vi "Teleop.vi"(10 "Match Info":T1={"Autonomous Elapsed Seconds"=0.0, "TeleOp Elapsed Seconds"=0.0, "Disabled Elapsed Seconds"=0.0, "Visited Autonomous"=FALSE, "Visited TeleOp"=FALSE, "Visited Disabled"=FALSE, "Autonomous Settings"={"Autonomous Style"=enum."Independent", "VI Refnum"=refnum}}, 11 "Call Context":T2) -> ()   [LabVIEW 2019]
doc: "This VI is called for each TeleOp packet received from the DS where the robot is not disabled. It is often used to read from the joysticks and update I/O or to update setpoints for timed control loops. It should complete and return within 20 milliseconds or it may miss DS packets."
uses:
  <vilib>/Rock Robotics/WPI/DriverStation/WPI_DriverStationDerivedRobotMode.ctl
  <vilib>/Rock Robotics/WPI/DriverStation/WPI_DriverStationMatch Info.ctl
  <vilib>/Rock Robotics/WPI/Utilities/WPI_GetSetVariantRefNum.vi
  <vilib>/Rock Robotics/Network Tables/NT Write Boolean Array.vi
  <vilib>/Rock Robotics/Network Tables/NT Write Numeric Array.vi
  <vilib>/Rock Robotics/Network Tables/NT Read Boolean.vi
  <vilib>/Rock Robotics/Network Tables/NT Read Number.vi
panel:
  out "Sample Slider 0":dbl(slide) scale=0.0..5.0
  out "Sample Boolean 1":bool
  out "Sample Boolean 0":bool
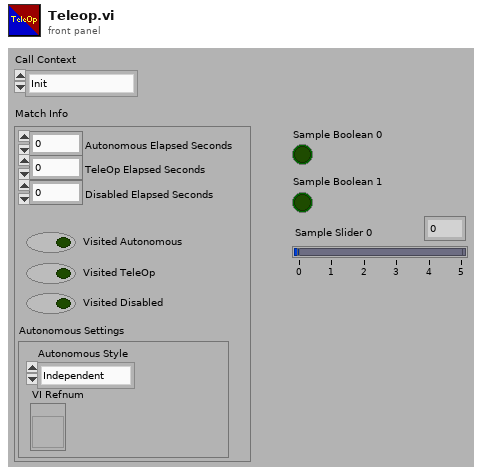
[diagram p1: front panel]
types:
  T1 = typedef "WPI_DriverStationMatch Info.ctl" = cluster{"Autonomous Elapsed Seconds":dbl, "TeleOp Elapsed Seconds":dbl, "Disabled Elapsed Seconds":dbl, "Visited Autonomous":bool, "Visited TeleOp":bool, "Visited Disabled":bool, "Autonomous Settings":cluster{"Autonomous Style":enum16{"Iterative", "Independent"}, "VI Refnum":refnum<vi>}}
  T2 = typedef "WPI_DriverStationDerivedRobotMode.ctl" = enum16{"Init", "Execute", "Stop"}
  T3 = typedef "WPI_JoystickDevRef.ctl" = cluster{"Device":T4}
  T4 = typedef "WPI_JoystickDeviceEnum.ctl" = enum16{"USB 0", "USB 1", "USB 2", "USB 3", "USB 4", "USB 5"}
  T5 = cluster{"Buttons[0]":bool, "Buttons[1]":bool, "Buttons[2]":bool, "Buttons[3]":bool, "Buttons[4]":bool, "Buttons[5]":bool, "Buttons[6]":bool, "Buttons[7]":bool, "Buttons[8]":bool}
  T6 = cluster{"Axes[0]":dbl, "Axes[1]":dbl, "Axes[2]":dbl, "Axes[3]":dbl, "Axes[4]":dbl, "Axes[5]":dbl, "Axes[6]":dbl, "Axes[7]":dbl, "Axes[8]":dbl}
  T7 = typedef "WPI_RobotDriveDevRef.ctl" = cluster{"DevStatus":errorcluster, "Motors[]":T8[], "Square Inputs":bool, "Max Output":dbl}
  T8 = typedef "WPI_MotorControlDeviceRef.ctl" = cluster{"DeviceStatus":errorcluster, "Type":T9, "PWM":cluster{"PWM Channel":T10, "DeadBand":T11}, "CAN":cluster{"Device Number":u8, "SetOutput VI Ref":variant, "GetOutput VI Ref":variant, "Enable VI Ref":variant, "Disable VI Ref":variant, "Data":variant}, "Invert":bool, "DIO PWM":cluster{"PWM \"Enable\" Channel":T10, "DIOChannel":T12, "PWM Rate":dbl}}
  T9 = typedef "WPI_MotorControlType.ctl" = enum16{"PWM", "CAN", "DIO PWM"}
  T10 = typedef "FPGA_DIOPWMChannel.ctl" = enum8{"PWM 0", "PWM 1", "PWM 2", "PWM 3", "PWM 4", "PWM 5", "PWM 6", "PWM 7", "PWM 8", "PWM 9", "PWM MXP 0", "PWM MXP 1", "PWM MXP 2", "PWM MXP 3", "PWM MXP 4", "PWM MXP 5", "PWM MXP 6", "PWM MXP 7", "PWM MXP 8", "PWM MXP 9", "Invalid"}
  T11 = typedef "WPI_PWMDeadband.ctl" = cluster{"Name":string, "maxPositivePwm":i32, "minPositivePwm":i32, "centerPwm":i32, "maxNegativePwm":i32, "minNegativePwm":i32, "angularRange":u16}
  T12 = typedef "FPGA_DIOChannel.ctl" = enum8{"DIO 0", "DIO 1", "DIO 2", "DIO 3", "DIO 4", "DIO 5", "DIO 6", "DIO 7", "DIO 8", "DIO 9", "DIO MXP 0", "DIO MXP 1", "DIO MXP 2", "DIO MXP 3", "DIO MXP 4", "DIO MXP 5", "DIO MXP 6", "DIO MXP 7", "DIO MXP 8", "DIO MXP 9", "DIO MXP 10", "DIO MXP 11", "DIO MXP 12", "DIO MXP 13", "DIO MXP 14", "DIO MXP 15", "SPI Port CS1", "SPI Port CS2", "SPI Port CS3", "SPI Port MISO", "SPI Port MOSI", "Invalid"}
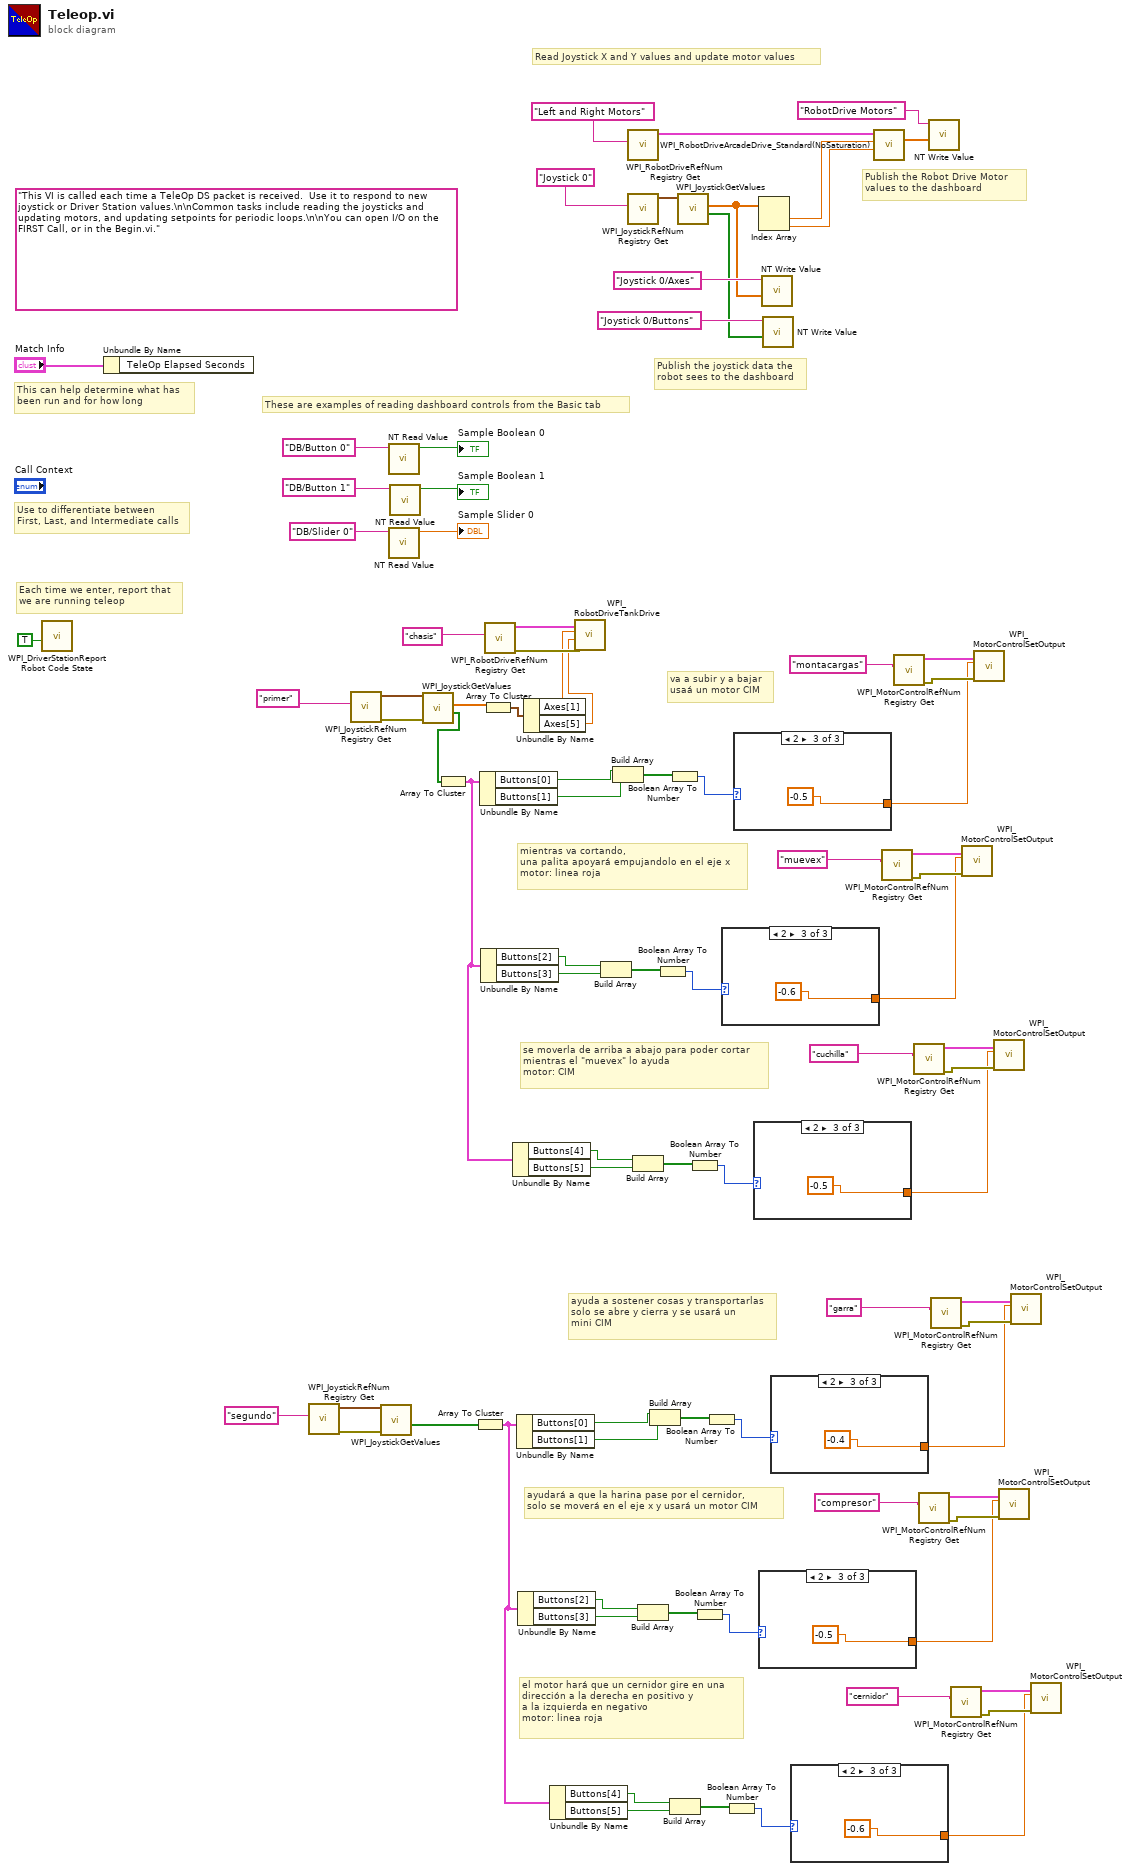
[diagram p0: block diagram]
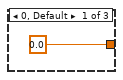
[diagram p2: hidden frame]
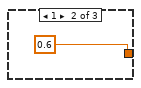
[diagram p3: hidden frame]
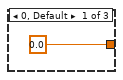
[diagram p4: hidden frame]
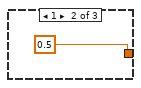
[diagram p5: hidden frame]
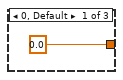
[diagram p6: hidden frame]
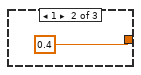
[diagram p7: hidden frame]
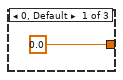
[diagram p8: hidden frame]
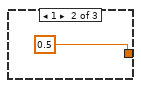
[diagram p9: hidden frame]
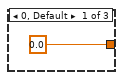
[diagram p10: hidden frame]
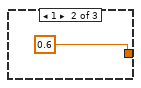
[diagram p11: hidden frame]
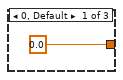
[diagram p12: hidden frame]
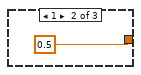
[diagram p13: hidden frame]
diagram:
  (unwired) "This VI is called each time a TeleOp DS packet is received.  Use it to respond to new joystick or Driver Station values.\n\nCommon tasks include reading the joysticks and updating motors, and updating setpoints for periodic loops.\n\nYou can open I/O on the FIRST Call, or in the Begin.vi."
  # "el motor hará que un cernidor gire en una\ndirección a la derecha en positivo y \na la izquierda en negativo\nmotor: linea roja"
  # "ayudará a que la harina pase por el cernidor,\nsolo se moverá en el eje x y usará un motor CIM"
  # "ayuda a sostener cosas y transportarlas\nsolo se abre y cierra y se usará un \nmini CIM"
  # "se moverla de arriba a abajo para poder cortar \nmientras el \"muevex\" lo ayuda\nmotor: CIM"
  # "mientras va cortando, \nuna palita apoyará empujandolo en el eje x\nmotor: linea roja"
  # "va a subir y a bajar\nusaá un motor CIM"
  # "These are examples of reading dashboard controls from the Basic tab"
  # "Publish the Robot Drive Motor\nvalues to the dashboard"
  # "Publish the joystick data the\nrobot sees to the dashboard"
  # "Each time we enter, report that\nwe are running teleop"
  # "Use to differentiate between\nFirst, Last, and Intermediate calls"
  # "This can help determine what has\nbeen run and for how long"
  # "Read Joystick X and Y values and update motor values"
  n1 = call <vilib>:"WPI_DriverStationReport Robot Code State.vi"("TeleOp"=TRUE ("Autonomous")) -> ()  [unwired: 10 in, 1 out]
  n2 = Unbundle By Name("Match Info") -> ()  [unwired: 1 out]
  n3 = call <vilib>:"WPI_JoystickRefNum Registry Get.vi"("refnum name"="segundo") -> ("error out"=w28:errorcluster, "JoystickDevRef"=w29:T3)  [unwired: 9 in]
  n4 = call <vilib>:"WPI_JoystickRefNum Registry Get.vi"("refnum name"="primer") -> ("error out"=w61:errorcluster, "JoystickDevRef"=w62:T3)  [unwired: 9 in]
  n5 = call <vilib>:"WPI_JoystickGetValues.vi"("error in (no error)"=w28, "JoystickDevRef"=w29) -> ("Buttons"=w27:bool[])  [unwired: 5 in, 4 out]
  n6 = call-poly <vilib>:"NT Read Value.vi"("Name"="DB/Button 0" ("refnum name")) -> ("Boolean"=→"Sample Boolean 0":bool)  [unwired: 9 in, 1 out]
  n7 = call-poly <vilib>:"NT Read Value.vi"("Name"="DB/Slider 0" ("refnum name")) -> ("Numeric"=→"Sample Slider 0":dbl)  [unwired: 9 in, 1 out]
  n8 = call-poly <vilib>:"NT Read Value.vi"("Name"="DB/Button 1" ("refnum name")) -> ("Boolean"=→"Sample Boolean 1":bool)  [unwired: 9 in, 1 out]
  n9 = call <vilib>:"WPI_JoystickGetValues.vi"("error in (no error)"=w61, "JoystickDevRef"=w62) -> ("Buttons"=w55:bool[], "Axes"=w59:dbl[])  [unwired: 5 in, 3 out]
  n10 = Array To Cluster(array=w55) -> (cluster=w30:T5)
  n11 = Array To Cluster(array=w27) -> (cluster=w2:T5)
  n12 = Unbundle By Name(w30) -> ("Buttons[0]"=w54:bool, "Buttons[1]"=w53:bool)
  n13 = Unbundle By Name(w30) -> ("Buttons[2]"=w40:bool, "Buttons[3]"=w39:bool)
  n14 = Array To Cluster(array=w59) -> (cluster=w58:T6)
  n15 = call <vilib>:"WPI_RobotDriveRefNum Registry Get.vi"("refnum name"="chasis") -> ("error out"=w65:errorcluster, "RobotDriveDevRef"=w64:T7)  [unwired: 9 in]
  n16 = Unbundle By Name(w30) -> ("Buttons[4]"=w32:bool, "Buttons[5]"=w31:bool)
  n17 = Unbundle By Name(w2) -> ("Buttons[0]"=w26:bool, "Buttons[1]"=w25:bool)
  n18 = Unbundle By Name(w2) -> ("Buttons[2]"=w12:bool, "Buttons[3]"=w11:bool)
  n19 = Unbundle By Name(w58) -> ("Axes[1]"=w57:dbl, "Axes[5]"=w56:dbl)
  n20 = Unbundle By Name(w2) -> ("Buttons[4]"=w4:bool, "Buttons[5]"=w3:bool)
  n21 = call <vilib>:"WPI_RobotDriveTankDrive.vi"("error in (no error)"=w65, "Right axis value"=w56, "Left axis value"=w57, "RobotDriveDevRef"=w64) -> ()  [unwired: 5 in, 3 out]
  n22 = Build Array(w40, w39) -> (w46:bool[])
  n23 = Build Array(w54, w53) -> (w52:bool[])
  n24 = call <vilib>:"WPI_RobotDriveRefNum Registry Get.vi"("refnum name"="Left and Right Motors") -> ("RobotDriveDevRef"=w83:T7)  [unwired: 1 in, 9 out]
  n25 = call <vilib>:"WPI_JoystickRefNum Registry Get.vi"("refnum name"="Joystick 0") -> ("JoystickDevRef"=w80:T3)  [unwired: 1 in, 9 out]
  n26 = Build Array(w32, w31) -> (w38:bool[])
  n27 = Build Array(w12, w11) -> (w18:bool[])
  n28 = Build Array(w26, w25) -> (w24:bool[])
  n29 = Boolean Array To Number(Boolean array=w46) -> (number=w45:u32)
  n30 = Boolean Array To Number(Boolean array=w52) -> (number=w51:u32)
  n31 = Build Array(w4, w3) -> (w10:bool[])
  n32 = call <vilib>:"WPI_JoystickGetValues.vi"("JoystickDevRef"=w80) -> ("Buttons"=w74:bool[], "Axes"=w75:dbl[])  [unwired: 6 in, 3 out]
  n33 = Boolean Array To Number(Boolean array=w38) -> (number=w37:u32)
  n34 = Boolean Array To Number(Boolean array=w18) -> (number=w17:u32)
  n35 = Boolean Array To Number(Boolean array=w24) -> (number=w23:u32)
  n36 = case shown="2" w45 {
    tunnel: [0.0 0.6 -0.6] -> w42
    frame 0, Default {
    }
    frame 1 {
    }
    frame 2 {
    }
  }
  n37 = Boolean Array To Number(Boolean array=w10) -> (number=w9:u32)
  n38 = case shown="2" w51 {
    tunnel: [0.0 0.5 -0.5] -> w48
    frame 0, Default {
    }
    frame 1 {
    }
    frame 2 {
    }
  }
  n39 = case shown="2" w37 {
    tunnel: [0.0 0.5 -0.5] -> w34
    frame 0, Default {
    }
    frame 1 {
    }
    frame 2 {
    }
  }
  n40 = Index Array(array=w75) -> (element #1=w82:dbl, element #2=w78:dbl)  [unwired: 2 in]
  n41 = case shown="2" w17 {
    tunnel: [0.0 0.5 -0.5] -> w14
    frame 0, Default {
    }
    frame 1 {
    }
    frame 2 {
    }
  }
  n42 = call-poly <vilib>:"NT Write Value.vi"("Numeric Array"=w75, "Name"="Joystick 0/Axes") -> ()  [unwired: 9 in, 1 out]
  n43 = call-poly <vilib>:"NT Write Value.vi"("Boolean Array"=w74, "Name"="Joystick 0/Buttons") -> ()  [unwired: 9 in, 1 out]
  n44 = case shown="2" w23 {
    tunnel: [0.0 0.4 -0.4] -> w20
    frame 0, Default {
    }
    frame 1 {
    }
    frame 2 {
    }
  }
  n45 = case shown="2" w9 {
    tunnel: [0.0 0.6 -0.6] -> w6
    frame 0, Default {
    }
    frame 1 {
    }
    frame 2 {
    }
  }
  n46 = call <vilib>:"WPI_RobotDriveArcadeDrive_Standard(NoSaturation).vi"("Y axis value"=w78, "X axis value"=w82, "RobotDriveDevRef"=w83) -> ("Motor Values"=w67:dbl[])  [unwired: 1 in, 7 out]
  n47 = call <vilib>:"WPI_MotorControlRefNum Registry Get.vi"("refnum name"="muevex") -> ("error out"=w43:errorcluster, "MotorControlDevRef"=w44:T8)  [unwired: 9 in]
  n48 = call <vilib>:"WPI_MotorControlRefNum Registry Get.vi"("refnum name"="montacargas") -> ("error out"=w49:errorcluster, "MotorControlDevRef"=w50:T8)  [unwired: 9 in]
  n49 = call <vilib>:"WPI_MotorControlRefNum Registry Get.vi"("refnum name"="cuchilla") -> ("error out"=w35:errorcluster, "MotorControlDevRef"=w36:T8)  [unwired: 9 in]
  n50 = call <vilib>:"WPI_MotorControlRefNum Registry Get.vi"("refnum name"="compresor") -> ("error out"=w15:errorcluster, "MotorControlDevRef"=w16:T8)  [unwired: 9 in]
  n51 = call-poly <vilib>:"NT Write Value.vi"("Numeric Array"=w67, "Name"="RobotDrive Motors") -> ()  [unwired: 9 in, 1 out]
  n52 = call <vilib>:"WPI_MotorControlRefNum Registry Get.vi"("refnum name"="garra") -> ("error out"=w21:errorcluster, "MotorControlDevRef"=w22:T8)  [unwired: 9 in]
  n53 = call <vilib>:"WPI_MotorControlRefNum Registry Get.vi"("refnum name"="cernidor") -> ("error out"=w7:errorcluster, "MotorControlDevRef"=w8:T8)  [unwired: 9 in]
  n54 = call <vilib>:"WPI_MotorControlSetOutput.vi"("error in (no error)"=w43, "Output"=w42, "MotorControlDevRef"=w44) -> ()  [unwired: 6 in, 3 out]
  n55 = call <vilib>:"WPI_MotorControlSetOutput.vi"("error in (no error)"=w49, "Output"=w48, "MotorControlDevRef"=w50) -> ()  [unwired: 6 in, 3 out]
  n56 = call <vilib>:"WPI_MotorControlSetOutput.vi"("error in (no error)"=w35, "Output"=w34, "MotorControlDevRef"=w36) -> ()  [unwired: 6 in, 3 out]
  n57 = call <vilib>:"WPI_MotorControlSetOutput.vi"("error in (no error)"=w15, "Output"=w14, "MotorControlDevRef"=w16) -> ()  [unwired: 6 in, 3 out]
  n58 = call <vilib>:"WPI_MotorControlSetOutput.vi"("error in (no error)"=w21, "Output"=w20, "MotorControlDevRef"=w22) -> ()  [unwired: 6 in, 3 out]
  n59 = call <vilib>:"WPI_MotorControlSetOutput.vi"("error in (no error)"=w7, "Output"=w6, "MotorControlDevRef"=w8) -> ()  [unwired: 6 in, 3 out]
